vi "Vecto Info Async.vi"(11 "VectoService in":refnum<class "VectoInfo.lvclass">) -> ()   [LabVIEW 2020, in "Vecto.lvlib" / "VectoInfo.lvclass"]
uses:
  VectoInfo.lvclass
  Loop Data.ctl
  Connection Info.ctl
  Connection Type.ctl
  Vecto Info.ctl
  VectoInfo.lvclass/VectoInfo.ctl
  VectoInfoValue/VectoInfoValue.lvclass/VectoInfoValue.ctl
  <vilib>/Utility/miscctls.llb/LVMapReplaceAction.ctl
  VectoInfoValue/VectoInfoValue.lvclass
  Vecto.lvlib
  lv-promises/Promises/Promise/Promise.lvclass
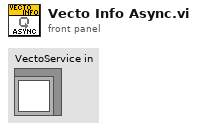
[diagram p1: front panel]
types:
  T1 = typedef "Vecto.lvlib/VectoInfo.lvclass/Loop Data.ctl" = cluster{"Connections":map{string, T2}, "Vecto Info":T4}
  T2 = typedef "Vecto.lvlib/Connection Info.ctl" = cluster{"Name":string, "Type":T3, "RXCount":i32, "TXCount":i32, "Connected":bool, "RemoteIP":u32, "RemotePort":u16, "LocalPort":u16, "Node ID":u32}
  T3 = typedef "Vecto.lvlib/Connection Type.ctl" = enum16{"TCP", "Telemetry", "Discovery", "HTTP"}
  T4 = typedef "Vecto.lvlib/Vecto Info.ctl" = cluster{"NodeID":i32, "IP":u32, "Connections":T2[]}
  T5 = typedef "LVMapReplaceAction.ctl" = enum32{"Modify Entry only if found", "Add or Modify Entry", "Delete Entry"}
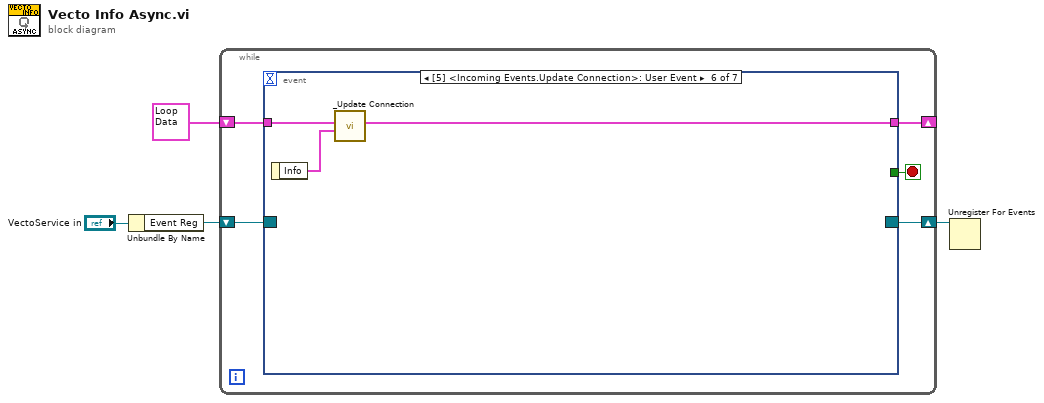
[diagram p0: block diagram]
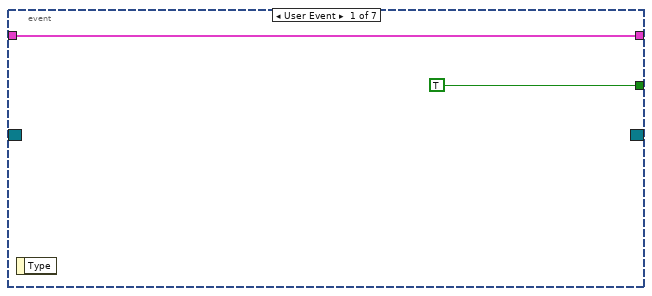
[diagram p2: hidden frame]
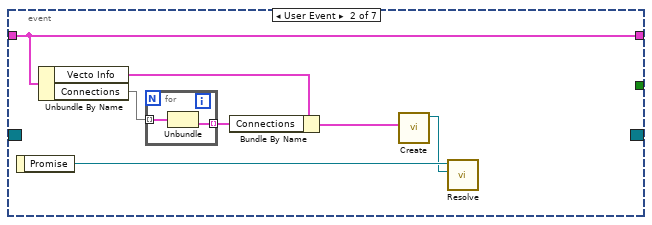
[diagram p3: hidden frame]
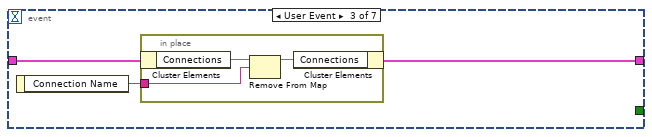
[diagram p4: hidden frame]
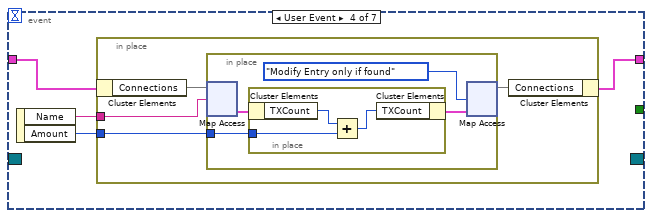
[diagram p5: hidden frame]
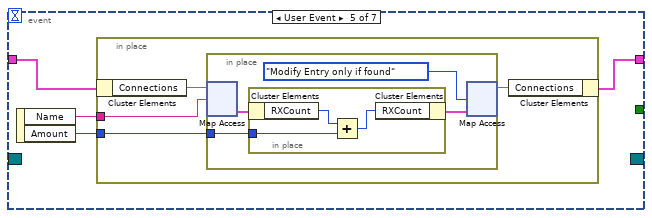
[diagram p6: hidden frame]
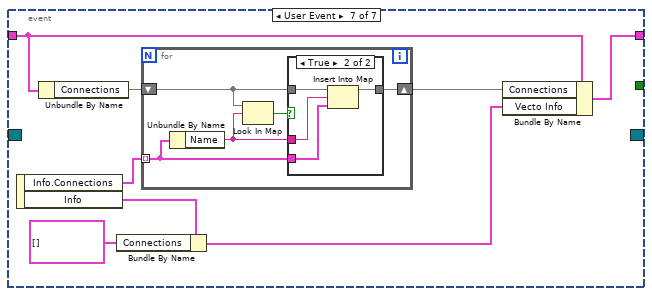
[diagram p7: hidden frame]
diagram:
  n1 = Unbundle By Name("VectoService in") -> ("Event Reg"=w2:refnum<event-registration>)
  n2 = while {
    shift-right: [w7] -> _
    shift-left: T1 {"Connections"={}, "Vecto Info"={"NodeID"=0, "IP"=0, "Connections"=[]}} ("Data") -> [w6]
    shift-right: [w8] -> w1
    shift-left: w2 -> [w9]
    stop <- w5 stop-if-true
    n3 = event shown="[5] <Incoming Events.Update Connection>: User Event" {
      selector: w9 -> [_ _ _ _ _ _ _]
      dyn-events: [_ _ _ _ _ _ _] -> w8
      timeout: _ -> [_ _ _ _ _ _ _]
      tunnel: [w11 w18 w21 w27 w42 w57 w61] -> w7
      tunnel: w6 -> [w11 w18 w23 w30 w45 w59 w60]
      tunnel: [TRUE _ _ _ _ _ _] -> w5
      event User Event {
        n4 = event-data() -> ()  [unwired: 1 in, 1 out]
      }
      event User Event {
        n5 = event-data() -> ("Promise"=w13:refnum<class "Promise.lvclass">)  [unwired: 1 in]
        n6 = Unbundle By Name(w18) -> ("Vecto Info"=w16:T4, "Connections"=w17:map{string, T2})
        n7 = for {
          tunnel: w17 -> [w20] mode=indexing
          tunnel: [w19] -> w15 mode=indexing
          n8 = Unbundle(w20) -> ("Info"=w19:T2)  [unwired: 1 out]
        }
        n9 = Bundle By Name(cluster=w16, "Connections"=w15) -> (w14:T4)
        n10 = call "Create.vi"("Vecto Info"=w14) -> ("VectoInfoValue out"=w12:refnum<class "VectoInfoValue.lvclass">)  [unwired: 10 in]
        n11 = call "Resolve.vi"("Result (None)"=w12, "Promise in"=w13) -> ()  [unwired: 8 in, 2 out]
      }
      event User Event {
        n12 = event-data() -> ("Connection Name"=w22:string)  [unwired: 1 in]
        n13 = in-place {
          in-place-border: w22 -> [w25]
          n14 = in-place-cluster #1(w23) -> ("Connections"=w26:map{string, T2})
          n15 = Remove From Map(10:w25, 11:w26) -> (3:w24:map{string, T2})  [unwired: 2 out]
          n16 = in-place-cluster #1("Connections"=w24) -> (w21:T1)
        }
      }
      event User Event {
        n17 = event-data() -> ("Name"=w29:string, "Amount"=w28:i32)  [unwired: 1 in]
        n18 = in-place {
          in-place-border: w29 -> [w33]
          in-place-border: w28 -> [w31]
          n19 = in-place-cluster #2(w30) -> ("Connections"=w34:map{string, T2})
          n20 = in-place {
            in-place-border: w31 -> [w36]
            n21 = in-place-map #3(w34, w33) -> (w38:T2)  [unwired: 1 in, 1 out]
            n22 = in-place {
              in-place-border: w36 -> [w40]
              n23 = in-place-cluster #4(w38) -> ("TXCount"=w41:i32)
              n24 = Add(x=w41, y=w40) -> (x+y=w39:i32)
              n25 = in-place-cluster #4("TXCount"=w39) -> (w37:T2)
            }
            n26 = in-place-map #3(w37, LVMapReplaceAction."Modify Entry only if found" ("action")) -> (w32:map{string, T2})  [unwired: 2 out]
          }
          n27 = in-place-cluster #2("Connections"=w32) -> (w27:T1)
        }
      }
      event User Event {
        n28 = event-data() -> ("Name"=w44:string, "Amount"=w43:i32)  [unwired: 1 in]
        n29 = in-place {
          in-place-border: w44 -> [w48]
          in-place-border: w43 -> [w46]
          n30 = in-place-cluster #5(w45) -> ("Connections"=w49:map{string, T2})
          n31 = in-place {
            in-place-border: w46 -> [w51]
            n32 = in-place-map #6(w49, w48) -> (w53:T2)  [unwired: 1 in, 1 out]
            n33 = in-place {
              in-place-border: w51 -> [w55]
              n34 = in-place-cluster #7(w53) -> ("RXCount"=w56:i32)
              n35 = Add(x=w56, y=w55) -> (x+y=w54:i32)
              n36 = in-place-cluster #7("RXCount"=w54) -> (w52:T2)
            }
            n37 = in-place-map #6(w52, LVMapReplaceAction."Modify Entry only if found" ("action")) -> (w47:map{string, T2})  [unwired: 2 out]
          }
          n38 = in-place-cluster #5("Connections"=w47) -> (w42:T1)
        }
      }
      event User Event {
        n39 = event-data() -> ("Info"=w58:T2)  [unwired: 1 in]
        n40 = call "_Update Connection.vi"("Info"=w58, "Data in"=w59) -> ("Data"=w57:T1)  [unwired: 8 in, 1 out]
      }
      event User Event {
        n41 = event-data() -> ("Info.Connections"=w64:T2[], "Info"=w67:T4)  [unwired: 1 in]
        n42 = Unbundle By Name(w60) -> ("Connections"=w65:map{string, T2})
        n43 = Bundle By Name(cluster=w67, "Connections"=T2[] []) -> (w62:T4)
        n44 = for {
          shift-right: [w68] -> w63
          shift-left: w65 -> [w69]
          tunnel: w64 -> [w71] mode=indexing
          n45 = Unbundle By Name(w71) -> ("Name"=w72:string)
          n46 = Look In Map(map=w69, key=w72) -> (key not found?=w70:bool)  [unwired: 1 in, 1 out]
          n47 = case shown="True" w70 {
            tunnel: w72 -> [_ w75]
            tunnel: w71 -> [_ w74]
            tunnel: w69 -> [w73 w77]
            tunnel: [w73 w76] -> w68
            frame False {
            }
            frame True {
              n48 = Insert Into Map(map in=w77, key=w75, value=w74) -> (map out=w76:map{string, T2})  [unwired: 2 out]
            }
          }
        }
        n49 = Bundle By Name(cluster=w60, "Connections"=w63, "Vecto Info"=w62) -> (w61:T1)
      }
    }
  }
  n50 = Unregister For Events(event registration refnum=w1) -> ()  [unwired: 1 in, 1 out]
